vi "StartClone.vi"(7 "ShowPanel? (f)":bool, 8 "error in (no error)":errorcluster, 10 "ModuleName":string="unnamed", 11 "vi path":path) -> (0 "error out":errorcluster, 1 "clAcPwrEvents":T1, 3 "ModuleAdmin":refnum<class "ModuleAdmin.lvclass">)   [LabVIEW 2018, in "AcPwrModule.lvlib"]
doc: "This VI launches Main.vi and returns a cluster of type definitions that can be used to send requests to Main.vi. The nomenclature \"clone\" is used in the title since numerous copies of Main.vi can be launched with this function."
uses:
  AcPwrModule.lvlib
  <userlib>/NIST/ModuleAdminLib/ModuleAdmin/ModuleAdmin.lvclass
  C:/Program Files (x86)/National Instruments/LabVIEW 2018/user.lib/NIST/ModuleAdminLib/ModuleAdminBase/ModuleAdminBase.lvclass
  AcPwrShared/AcPwrBroadcastEvents.ctl
  AcPwrShared/clEventType.ctl
  <userlib>/NIST/ModuleAdminLib/ModuleAdmin/ModuleAdmin.lvclass/ModuleAdmin.ctl
  <userlib>/NIST/ModuleAdminLib/ModuleAdmin/Accessors/Write ShowPanel_.vi
  <userlib>/NIST/ModuleAdminLib/ModuleAdmin/Accessors/Write CloneRegRef.vi
  <vilib>/Utility/error.llb/Error Cluster From Error Code.vi
  <vilib>/ErrorRing/Error Ring.xnode
  AcPwrShared/AcPwrShared.lvlib
  <userlib>/NIST/ModuleAdminLib/ModuleAdminBase/ModuleAdminBase.lvclass
  <userlib>/NIST/ModuleAdminLib/CloneRegistration/CloneRegistration.lvclass
panel:
  # "If you want to add another Broadcast Events, open this typedef, copy an existing event and rename it to your event name.\n\nNext create an \"arg\" typedef for the  data and put it into PublicAPI/Arguments/Broadcasts\n\nAfter that, you will need to create a new roadcast vi in Protected/Broadcast.  Look at DidInit.vi or the reportError.vi as examples."
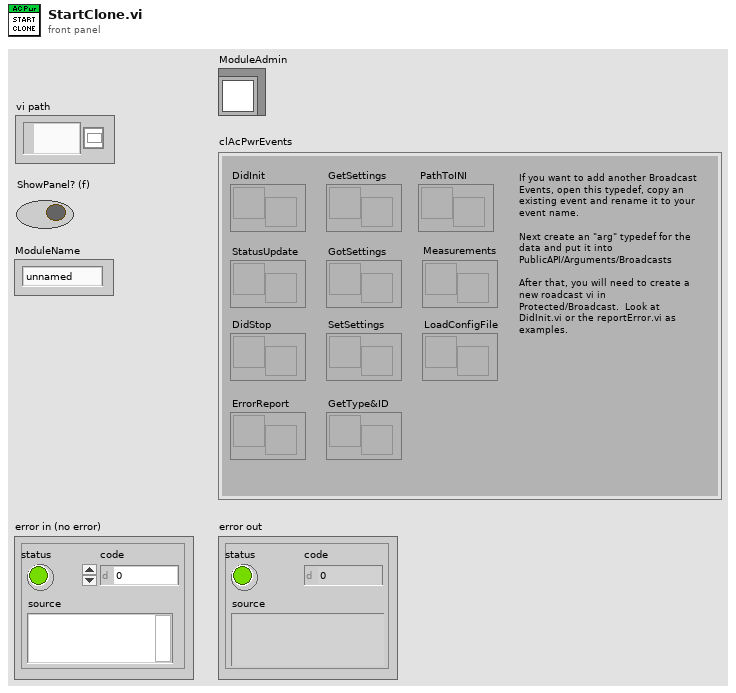
[diagram p1: front panel]
types:
  T1 = typedef "AcPwrShared.lvlib/AcPwrBroadcastEvents.ctl" = cluster{"DidInit":refnum<user-event>, "StatusUpdate":refnum<user-event>, "ErrorReport":refnum<user-event>, "DidStop":refnum<user-event>, "PathToINI":refnum<user-event>, "Measurements":refnum<user-event>, "LoadConfigFile":refnum<user-event>, "GetSettings":refnum<user-event>, "SetSettings":refnum<user-event>, "GetType&ID":refnum<user-event>, "GotSettings":refnum<user-event>}
  T2 = enum32{"Bad", "Idle", "Run top level", "Running"}
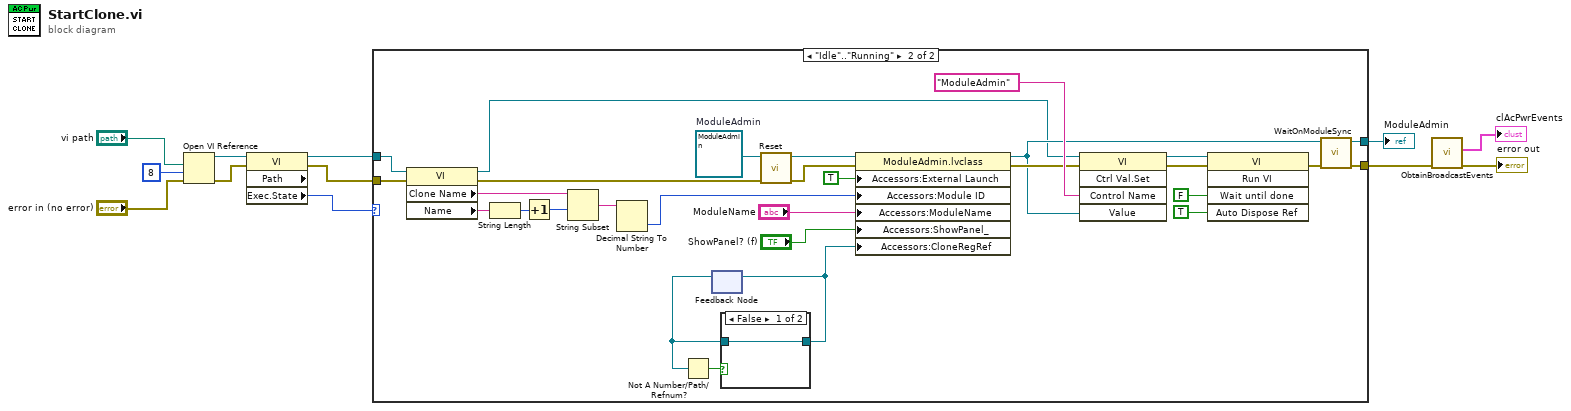
[diagram p0: block diagram]
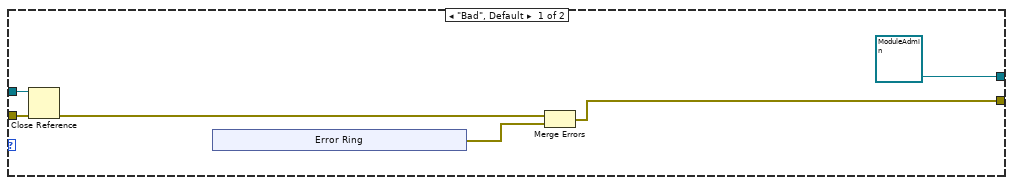
[diagram p2: hidden frame]
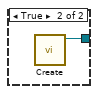
[diagram p3: hidden frame]
diagram:
  n1 = Open VI Reference(vi path="vi path", options=8, error in (no error)="error in (no error)") -> (vi reference=w4:refnum<vi>, error out=w5:errorcluster)  [unwired: 3 in]
  n2 = property class="VI" props=["Path", "Exec.State"](reference=w4, error in=w5) -> (reference out=w3:refnum<vi>, error out=w6:errorcluster, "Exec.State"=w12:T2)  [unwired: 1 out]
  n3 = case shown="\"Idle\"..\"Running\"" w12 {
    tunnel: w6 -> [w18 w29]
    tunnel: w3 -> [w17 w43]
    tunnel: [w14 w34] -> w11
    tunnel: [refnum<class "ModuleAdmin.lvclass"> refnum ("ModuleAdmin") w33] -> w9
    frame "Bad", Default {
      n4 = Close Reference(reference=w17, error in (no error)=w18) -> (error out=w16:errorcluster)
      n5 = xnode "Error Ring"() -> ("error out"=w15:errorcluster)
      n6 = Merge Errors(w16, w15) -> (w14:errorcluster)
    }
    frame "Idle".."Running" {
      w46 = refnum<class "ModuleAdmin.lvclass"> refnum  # ModuleAdmin
      n7 = property class="VI"(reference=w43, error in=w29) -> (reference out=w28:refnum<vi>, error out=w27:errorcluster, "Clone Name"=w48:string, "Name"=w51:string)
      n8 = String Length(string=w51) -> (length=w50:i32)
      n9 = Increment(x=w50) -> (x+1=w49:i32)
      n10 = String Subset(string=w48, offset (0)=w49) -> (substring=w47:string)  [unwired: 1 in]
      n11 = Decimal String To Number(string=w47) -> (number=w23:i32)  [unwired: 2 in, 1 out]
      n12 = feedback #1() -> (w30:refnum<data-value>)  [unwired: 1 in]
      n13 = Not A Number/Path/Refnum?(number/path/refnum=w30) -> (NaN/Path/Refnum?=w31:bool)
      n14 = case shown="False" w31 {
        tunnel: [w52 w53] -> w25
        tunnel: w30 -> [w52 _]
        frame False {
        }
        frame True {
          n15 = call <userlib>:"Create.vi"() -> ("CloneRegRef"=w53:refnum<data-value>)  [unwired: 10 in, 1 out]
        }
      }
      n16 = feedback-in #1(w25) -> ()
      n17 = call <userlib>:"Reset.vi"("error in (no error)"=w27, "Mod Admin in"=w46) -> ("error out"=w45:errorcluster, "Mod Admin out"=w44:refnum<class "ModuleAdmin.lvclass">)  [unwired: 8 in]
      n18 = property class="ModuleAdmin.lvclass"(reference=w44, error in=w45, "Accessors:External Launch"=TRUE ("External Launch"), "Accessors:Module ID"=w23, "Accessors:ModuleName"="ModuleName", "Accessors:ShowPanel_"="ShowPanel? (f)", "Accessors:CloneRegRef"=w25) -> (reference out=w35:refnum<class "ModuleAdmin.lvclass">, error out=w36:errorcluster)
      n19 = invoke class="VI" method="Ctrl Val.Set"(reference=w28, error in=w36, "Control Name"="ModuleAdmin", "Value"=w35) -> (reference out=w41:refnum<vi>, error out=w40:errorcluster)  [unwired: 1 in, 3 out]
      n20 = invoke class="VI" method="Run VI"(reference=w41, error in=w40, "Wait until done"=FALSE ("Wait Until Done"), "Auto Dispose Ref"=TRUE ("Auto Dispose Reference")) -> (error out=w37:errorcluster)  [unwired: 1 in, 4 out]
      n21 = call <userlib>:"WaitOnModuleSync.vi"("error in (no error)"=w37, "ModuleAdmin"=w35) -> ("error out"=w34:errorcluster, "ModuleAdmin"=w33:refnum<class "ModuleAdmin.lvclass">)  [unwired: 8 in]
    }
  }
  "ModuleAdmin" <- w9
  n22 = call "ObtainBroadcastEvents.vi"("error in (no error)"=w11) -> ("error out"=→"error out":errorcluster, "clAcPwrEvents"=→"clAcPwrEvents":T1)  [unwired: 9 in]
